vi "Read ECID File.vi"(8 "error in":errorcluster) -> (0 "error out":errorcluster, 3 "ECID Data":T1[](array[typedef]))   [LabVIEW 2020, in "SECS Communication.lvlib" / "SECS Data Class.lvclass"]
uses:
  SECS Data Class.lvclass
  ECID Data.ctl
  SECS-II Class/Format Code.ctl
  <vilib>/DATA AHEAD/XLR8/functions/Workbook/Open Create Workbook XLSX.vi
  <vilib>/DATA AHEAD/XLR8/XLR8.lvlib
  SECS-II Class/SECS-II Class.lvclass
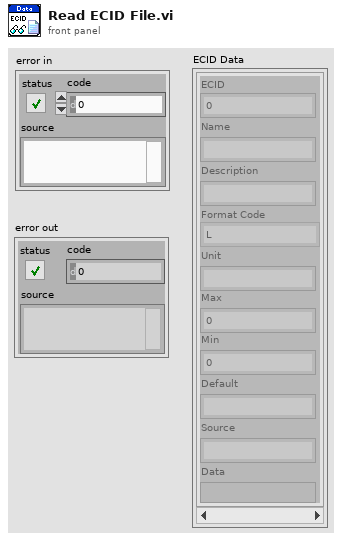
[diagram p1: front panel]
types:
  T1 = typedef "SECS Communication.lvlib/SECS Data Class.lvclass/ECID Data.ctl" = cluster{"ECID":u32, "Name":string, "Description":string, "Format Code":T2, "Unit":string, "Max":dbl, "Min":dbl, "Default":string, "Source":string, "Data":variant}
  T2 = typedef "SECS Communication.lvlib/SECS-II Class.lvclass/Format Code.ctl" = enum16{"L", "A", "B", "Boolean", "J", "I1", "I2", "I4", "I8", "U1", "U2", "U4", "U8", "F4", "F8", "Char"}
  T3 = typedef "XLR8.lvlib/XLR8_Ref.ctl" = cluster{"WBK":refnum<k24>, "CurSheet":refnum<k24>, "File":refnum<k24>, "file path":string, "sheet":string, "Sheets":refnum<k24>[], "IsXML":bool, "Policy":i32}
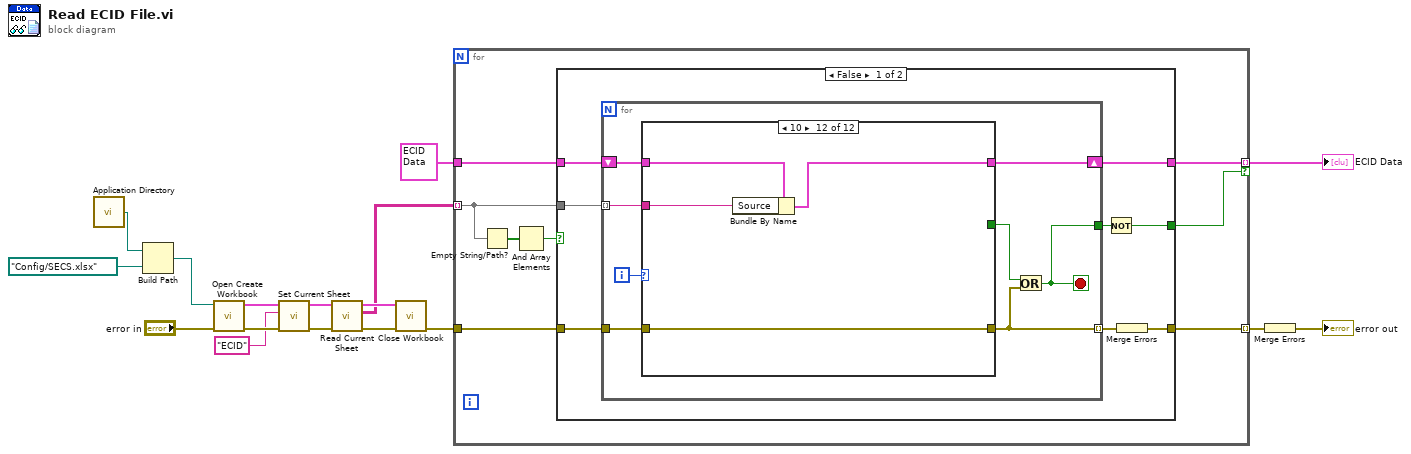
[diagram p0: block diagram]
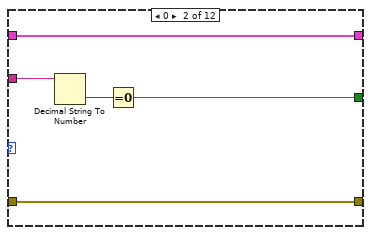
[diagram p3: hidden frame]
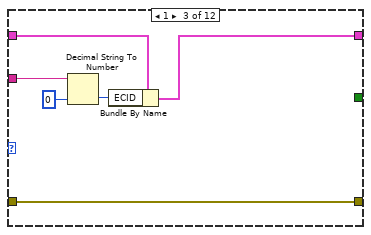
[diagram p4: hidden frame]
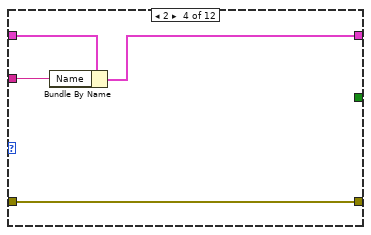
[diagram p5: hidden frame]
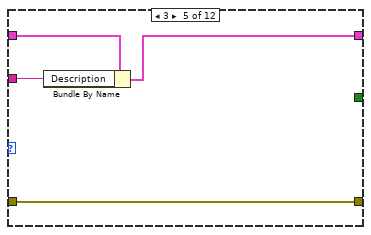
[diagram p6: hidden frame]
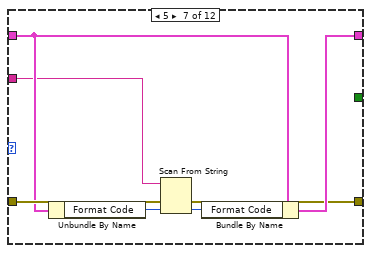
[diagram p8: hidden frame]
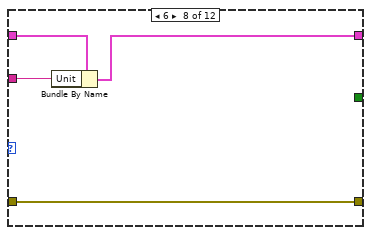
[diagram p9: hidden frame]
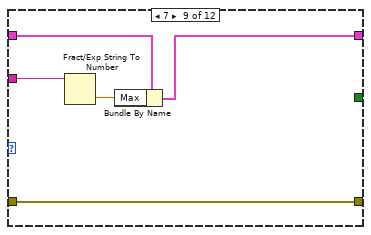
[diagram p10: hidden frame]
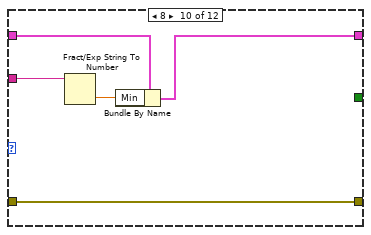
[diagram p11: hidden frame]
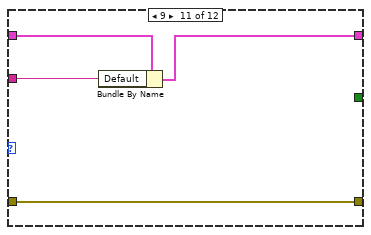
[diagram p12: hidden frame]
diagram:
  n1 = call <vilib>:"Application Directory.vi"() -> ("Application Directory"=w17:path)
  n2 = Build Path(base path=w17, name or relative path=path "Config/SECS.xlsx") -> (appended path=w14:path)
  n3 = call-poly <vilib>:"Open Create Workbook.vi"("error in"="error in", "Workbook Path"=w14) -> ("error out"=w12:errorcluster, "Refs Out"=w13:T3)  [unwired: 8 in]
  n4 = call <vilib>:"Set Current Sheet.vi"("error in"=w12, "Sheet to switch to"="ECID", "Refs In"=w13) -> ("error out"=w9:errorcluster, "Refs Out"=w10:T3)  [unwired: 7 in]
  n5 = call <vilib>:"Read Current Sheet.vi"("error in"=w9, "Refs In"=w10) -> ("error out"=w7:errorcluster, "Sheet-data out"=w5:string[][], "Refs Out"=w8:T3)  [unwired: 7 in]
  n6 = call <vilib>:"Close Workbook.vi"("error in"=w7, "Refs In"=w8) -> ("error out"=w6:errorcluster)  [unwired: 8 in, 1 out]
  n7 = for {
    tunnel: w6 -> [w22]
    tunnel: w5 -> [w23] mode=indexing
    tunnel: T1 {"ECID"=0, "Name"="", "Description"="", "Format Code"=enum."L", "Unit"="", "Max"=0.0, "Min"=0.0, "Default"="", "Source"="", "Data"=variant} ("ECID Data") -> [w21]
    tunnel: [w20] -> w1 mode=indexing if=w19
    tunnel: [w18] -> w4 mode=indexing
    n8 = Empty String/Path?(string/path=w23) -> (empty?=w25:bool[])
    n9 = And Array Elements(Boolean array=w25) -> (logical AND=w24:bool)
    n10 = case shown="False" w24 {
      tunnel: w23 -> [w33 _]
      tunnel: w22 -> [w28 w94]
      tunnel: w21 -> [w32 w95]
      tunnel: [w31 w95] -> w20
      tunnel: [w29 _] -> w19
      tunnel: [w26 w94] -> w18
      frame False {
        n11 = for {
          tunnel: w33 -> [w39] mode=indexing
          shift-right: [w38] -> w31
          shift-left: w32 -> [w41]
          tunnel: [w34] -> w30
          tunnel: w28 -> [w37]
          tunnel: [w35] -> w27 mode=indexing
          i -> [w40]
          stop <- w34 stop-if-true
          n12 = case shown="10" w40 {
            tunnel: w41 -> [w43 w48 w54 w58 w62 w64 w69 w74 w79 w84 w88 w92]
            tunnel: w39 -> [_ w47 w53 w57 w61 _ w67 w73 w77 w82 w86 w90]
            tunnel: [w43 w48 w50 w56 w60 w64 w71 w75 w80 w85 w89 w93] -> w38
            tunnel: [_ w45 _ _ _ _ _ _ _ _ _ _] -> w36
            tunnel: w37 -> [w42 w44 w49 w55 w59 w63 w70 w72 w78 w83 w87 w91]
            tunnel: [w42 w44 w49 w55 w59 w63 w65 w72 w78 w83 w87 w91] -> w35
            frame Default {
            }
            frame 0 {
              n13 = Decimal String To Number(string=w47) -> (number=w46:i32)  [unwired: 2 in, 1 out]
              n14 = Equal To 0?(x=w46) -> (x = 0?=w45:bool)
            }
            frame 1 {
              n15 = Decimal String To Number(string=w53, default (0L)=u32 0 ("default (0 I32)")) -> (number=w52:u32)  [unwired: 1 in, 1 out]
              n16 = Bundle By Name(cluster=w54, "ECID"=w52) -> (w50:T1)
            }
            frame 2 {
              n17 = Bundle By Name(cluster=w58, "Name"=w57) -> (w56:T1)
            }
            frame 3 {
              n18 = Bundle By Name(cluster=w62, "Description"=w61) -> (w60:T1)
            }
            frame 4 {
            }
            frame 5 {
              n19 = Unbundle By Name(w69) -> ("Format Code"=w68:T2)
              n20 = Scan From String(input string=w67, error in=w70, default 1=w68) -> (error out=w65:errorcluster, output 1=w66:T2)  [unwired: 2 in, 2 out]
              n21 = Bundle By Name(cluster=w69, "Format Code"=w66) -> (w71:T1)
            }
            frame 6 {
              n22 = Bundle By Name(cluster=w74, "Unit"=w73) -> (w75:T1)
            }
            frame 7 {
              n23 = Fract/Exp String To Number(string=w77) -> (number=w76:dbl)  [unwired: 3 in, 1 out]
              n24 = Bundle By Name(cluster=w79, "Max"=w76) -> (w80:T1)
            }
            frame 8 {
              n25 = Fract/Exp String To Number(string=w82) -> (number=w81:dbl)  [unwired: 3 in, 1 out]
              n26 = Bundle By Name(cluster=w84, "Min"=w81) -> (w85:T1)
            }
            frame 9 {
              n27 = Bundle By Name(cluster=w88, "Default"=w86) -> (w89:T1)
            }
            frame 10 {
              n28 = Bundle By Name(cluster=w92, "Source"=w90) -> (w93:T1)
            }
          }
          n29 = Or(x=w36, y=w35) -> (x .or. y?=w34:bool)
        }
        n30 = Not(x=w30) -> (.not. x?=w29:bool)
        n31 = Merge Errors(w27) -> (w26:errorcluster)
      }
      frame True {
      }
    }
  }
  "ECID Data" <- w1
  n32 = Merge Errors(w4) -> (→"error out":errorcluster)
